vi "GET_Location-based_density_map.vi"(0 "ImageSize":cluster{"x":i32, "y":i32}, 1 "Input array is image? (F)":bool, 5 "XY data":cluster{"Numeric":dbl, "Numeric":dbl}[](array[cluster]), 7 "Log2-transform? (T)":bool=TRUE, 9 "Normalize to 8 bit? (T)":bool=TRUE, 11 "error in (no error)":errorcluster, 12 "Output as Image? (F)":bool) -> (4 "Array or 8-bit pixmap out":u32[][](array[numeric]), 15 "error out":errorcluster)   [LabVIEW 2018, in "Tracker.lvlib"]
uses:
  Tracker.lvlib
  Controls/CTL_2D_bins_parameters.ctl
  GET_2D_Data_Binning_(location).vi
panel:
  out "Interp. size":i32[](array[numeric])
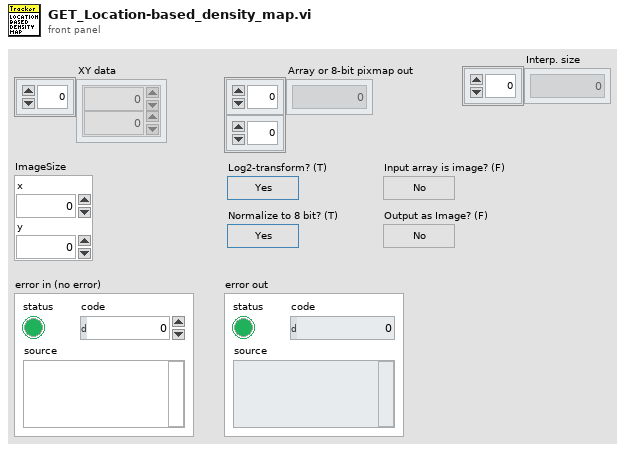
[diagram p1: front panel]
types:
  T1 = typedef "Tracker.lvlib/CTL_2D_bins_parameters.ctl" = cluster{"Xmax":dbl, "Xmin":dbl, "Ymax":dbl, "Ymin":dbl, "# bins per axis":i32}
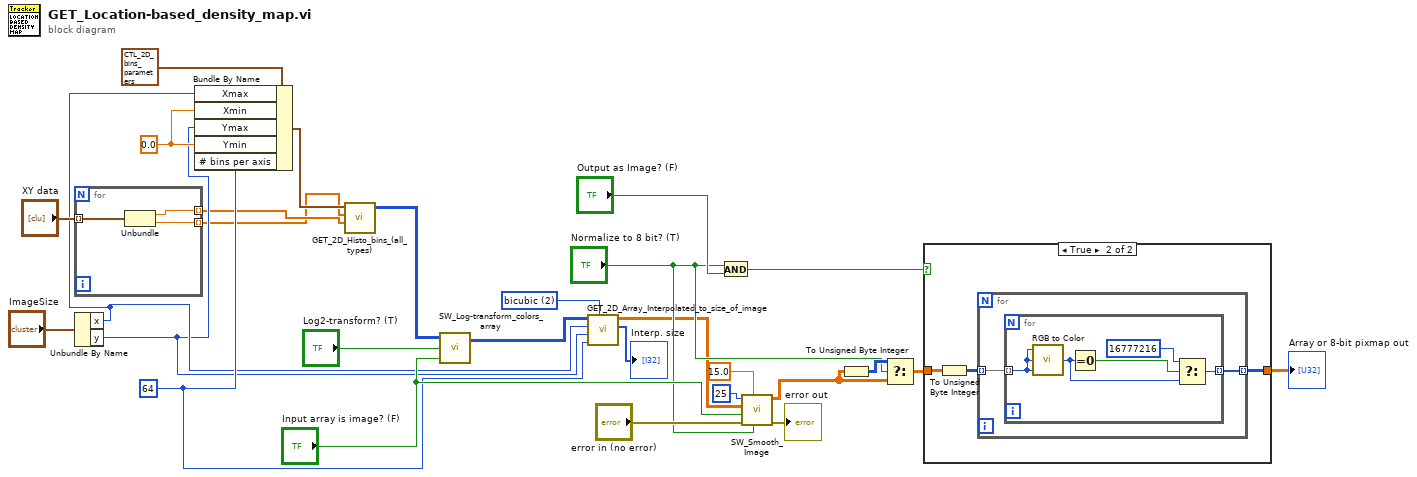
[diagram p0: block diagram]
diagram:
  w17 = 2 items=["nearest", "bilinear", "bicubic", "bicubic spline"] ("Method")
  w16 = 64 ("# bins per axis")
  w21 = 0.0 ("Xmin")
  n1 = for {
    tunnel: "XY data" -> [w31] mode=indexing
    tunnel: [w30] -> w2 mode=indexing
    tunnel: [w29] -> w1 mode=indexing
    n2 = Unbundle(w31) -> ("Numeric"=w30:dbl, "Numeric"=w29:dbl)
  }
  n3 = Unbundle By Name("ImageSize") -> ("x"=w4:i32, "y"=w3:i32)
  n4 = Bundle By Name(cluster=T1 {"Xmax"=110.0, "Xmin"=-110.0, "Ymax"=110.0, "Ymin"=-110.0, "# bins per axis"=64} ("Bins parameters"), "Xmax"=w4, "Xmin"=w21, "Ymax"=w3, "Ymin"=w21, "# bins per axis"=w16) -> (w22:T1)
  n5 = call-poly "GET_2D_Histo_bins_(all_types).vi"("Y"=w2, "X"=w1, "Bins parameters"=w22) -> ("Binned array"=w8:u32[][])  [unwired: 3 in]
  n6 = call "SW_Log-transform_colors_array.vi"("Image? (T)"="Input array is image? (F)", "Log-transform? (F)"="Log2-transform? (T)", "Array or 24-bit pixmap in"=w8) -> ("Array or 24-bit pixmap out"=w7:u32[][])  [unwired: 1 in]
  n7 = call "GET_2D_Array_Interpolated_to_size_of_image.vi"("Method"=w17, "# bins per axis"=w16, "Y image size"=w3, "X image size"=w4, "Array or pixmap in"=w7) -> ("Interp. size"=→"Interp. size":i32[], "Array or pixmap out"=w6:dbl[][])  [unwired: 5 in]
  n8 = And(x="Normalize to 8 bit? (T)", y="Output as Image? (F)") -> (x .and. y?=w10:bool)
  n9 = call "SW_Smooth_Image.vi"("Normalize? (T)"="Normalize to 8 bit? (T)", "Sigma"=15.0, "Error In"="error in (no error)", "Image? (T)"="Input array is image? (F)", "Array or pixmap in"=w6, "Kernel size"=u32 25) -> ("Error Out"=→"error out":errorcluster, "Array or pixmap out"=w5:dbl[][])  [unwired: 4 in]
  n10 = To Unsigned Byte Integer(number=w5) -> (unsigned 8bit integer=w14:u8[][])
  n11 = Select(t=w14, s="Normalize to 8 bit? (T)", f=w5) -> (s? t:f=w11:dbl[][])
  n12 = case shown="True" w10 {
    tunnel: [w32 w34] -> w12
    tunnel: w11 -> [w32 w35]
    frame False {
    }
    frame True {
      n13 = To Unsigned Byte Integer(number=w35) -> (unsigned 8bit integer=w33:u8[][])
      n14 = for {
        tunnel: w33 -> [w37] mode=indexing
        tunnel: [w36] -> w34 mode=indexing
        n15 = for {
          tunnel: w37 -> [w42] mode=indexing
          tunnel: [w41] -> w36 mode=indexing
          n16 = call <vilib>:"RGB to Color.vi"("B"=w42, "G"=w42, "R"=w42) -> ("Color"=w39:u32)
          n17 = Equal To 0?(x=w39) -> (x = 0?=w40:bool)
          n18 = Select(t=16777216, s=w40, f=w39) -> (s? t:f=w41:u32)
        }
      }
    }
  }
  "Array or 8-bit pixmap out" <- w12
